vi "Begin_FlyWheel.vi"() -> (0 "error out":errorcluster)   [LabVIEW 2012]
doc: "Called before other user functions, this VI is expected to open initial I/O refnums, load in file data, and do all program initialization. Notice that the <B>error out</B> terminal is simply used for data flow. Wiring it to other structures or subVIs ensures that this VI runs first."
uses:
  <vilib>/Rock Robotics/WPI/CAN/Jaguar/SubVIs/WPI_CANJaguar_ControlMode.ctl
  <vilib>/Rock Robotics/WPI/CAN/Jaguar/SubVIs/WPI_CANJaguar_SpeedReference.ctl
  <vilib>/Rock Robotics/WPI/CAN/Jaguar/SubVIs/WPI_CANJaguar_BrakeCoastMode.ctl
  <vilib>/Rock Robotics/WPI/MotorControl/WPI_MotorControlOpenCANJaguar.vi
panel:
  out "Succeeded?":bool
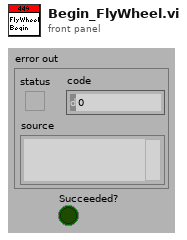
[diagram p1: front panel]
types:
  T1 = typedef "WPI_CANJaguar_BrakeCoastMode.ctl" = enum8{"Jumper", "Brake", "Coast"}
  T2 = typedef "WPI_CANJaguar_SpeedReference.ctl" = u8
  T3 = typedef "WPI_CANJaguar_ControlMode.ctl" = enum8{"Percent VBus", "Current", "Speed", "Position", "Voltage"}
  T4 = typedef "WPI_MotorControlDeviceRef.ctl" = cluster{"DeviceStatus":errorcluster, "Type":enum16{"PWM", "CAN"}, "PWM":cluster{"Digital Module":T5, "PWM Channel":T6, "DeadBand":T7}, "CAN":cluster{"Device Number":u8, "Control Mode":T3, "Semaphore":T8, "Max Vout":dbl}, "Invert":bool, "TransformRef":T9, "InvTransformRef":T9}
  T5 = typedef "FPGA_TypedefDigitalModule.ctl" = enum16{"Digital Module 1", "Digital Module 2"}
  T6 = typedef "FPGA_DIOPWMChannel.ctl" = enum8{"PWM 1", "PWM 2", "PWM 3", "PWM 4", "PWM 5", "PWM 6", "PWM 7", "PWM 8", "PWM 9", "PWM 10", "Invalid"}
  T7 = typedef "WPI_PWMDeadband.ctl" = cluster{"Name":string, "maxPositivePwm":i32, "minPositivePwm":i32, "centerPwm":i32, "maxNegativePwm":i32, "minNegativePwm":i32, "angularRange":u16}
  T8 = typedef "Semaphore RefNum" = refnum<k1>
  T9 = typedef "WPI_PWMTransform_ConPane.ctl" = refnum<vi>
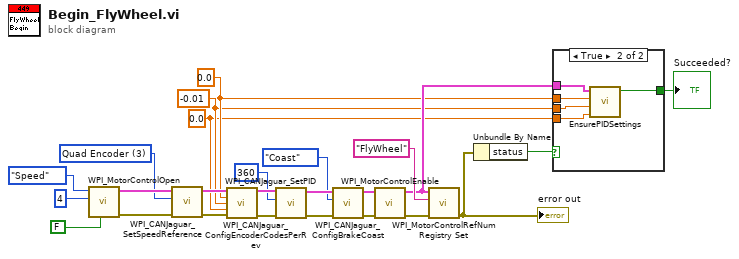
[diagram p0: block diagram]
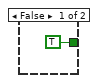
[diagram p2: hidden frame]
diagram:
  w4 = 0.0 ("P")
  w3 = -0.01 ("I")
  w2 = 0.0 ("D")
  w22 = T2 3 items=["Encoder"=0, "Inv Encoder"=2, "Quad Encoder"=3, "None"=255] ("Speed Reference")
  n1 = call-poly <vilib>:"WPI_MotorControlOpen.vi"("Invert"=FALSE, "Device Number"=u8 4, "Control Mode"=WPI_CANJaguar_ControlMode."Speed") -> ("error out"=w19:errorcluster, "MotorControlDeviceRef"=w23:T4)  [unwired: 7 in]
  n2 = call <vilib>:"WPI_CANJaguar_SetSpeedReference.vi"("error in (no error)"=w19, "Speed Reference"=w22, "CAN Jaguar Ref"=w23) -> ("error out"=w18:errorcluster, "CAN Jaguar Ref Out"=w21:T4)  [unwired: 7 in]
  n3 = call <vilib>:"WPI_CANJaguar_SetPID.vi"("CAN Jaguar Ref"=w21, "P"=w4, "I"=w3, "D"=w2, "error in (no error)"=w18) -> ("CAN Jaguar Ref Out"=w15:T4, "error out"=w16:errorcluster)  [unwired: 9 in]
  n4 = call <vilib>:"WPI_CANJaguar_ConfigEncoderCodesPerRev.vi"("error in (no error)"=w16, "Encoder Codes Per Rev"=u16 360, "CAN Jaguar Ref"=w15) -> ("error out"=w10:errorcluster, "CAN Jaguar Ref Out"=w13:T4)  [unwired: 7 in]
  n5 = call <vilib>:"WPI_CANJaguar_ConfigBrakeCoast.vi"("error in (no error)"=w10, "Brake / Coast Mode"=WPI_CANJaguar_BrakeCoastMode."Coast", "CAN Jaguar Ref"=w13) -> ("error out"=w11:errorcluster, "CAN Jaguar Ref Out"=w12:T4)  [unwired: 7 in]
  n6 = call <vilib>:"WPI_MotorControlEnable.vi"("error in (no error)"=w11, "CAN Jaguar Ref"=w12) -> ("error out"=w17:errorcluster, "CAN Jaguar Ref Out"=w5:T4)  [unwired: 8 in]
  n7 = call <vilib>:"WPI_MotorControlRefNum Registry Set.vi"("error in (no error)"=w17, "refnum name"="FlyWheel", "MotorControlDevRef"=w5) -> ("error out"=w7:errorcluster)  [unwired: 7 in, 1 out]
  "error out" <- w7
  n8 = Unbundle By Name(w7) -> ("status"=w6:bool)
  n9 = case shown="True" w6 {
    tunnel: w5 -> [_ w31]
    tunnel: w4 -> [_ w30]
    tunnel: w3 -> [_ w29]
    tunnel: w2 -> [_ w28]
    tunnel: [TRUE ("Succeeded?") w27] -> w1
    frame False {
    }
    frame True {
      n10 = call "EnsurePIDSettings.vi"("D"=w28, "I"=w29, "P"=w30, "CAN Jaguar Ref"=w31) -> ("Succeeded?"=w27:bool)  [unwired: 7 in]
    }
  }
  "Succeeded?" <- w1
